vi "PWM Panel.vi"(8 "error in (no error)":errorcluster, 9 "PWM Configuration (\"\")":string, 10 "PWM Stimulus":T3={"Zero"=FALSE, "Blank Screen"=FALSE, "Offset"=FALSE, "Offset Value"=4.0, "Frequency (MHz)"=0.0}, 11 "PWM Command":T1=enum."MEASURE") -> (0 "error out":errorcluster, 1 "Variant Output":string, 2 "PWM Measurement":T2 caption="This reading is always in the base units\ni.e. V, A, Ohms, Hz, Sec, etc." format="%#_10f")   [LabVIEW 2011]
uses:
  PWM Measurement.ctl
  PWM Parameters.ctl
  PWM Command.ctl
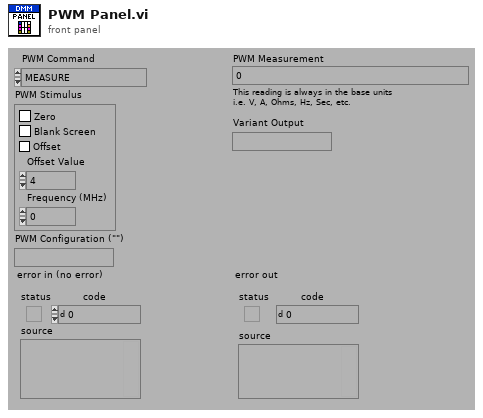
[diagram p1: front panel]
types:
  T1 = typedef "PWM Command.ctl" = enum16{"LOAD", "INITIALIZE", "PRESET", "GET STIMULUS", "SET STIMULUS", "MEASURE", "RELEASE", "UNLOAD", "GET CALIBRATION", "CALIBRATE"}
  T2 = typedef "PWM Measurement.ctl" = dbl
  T3 = typedef "PWM Parameters.ctl" = cluster{"Zero":bool, "Blank Screen":bool, "Offset":bool, "Offset Value":dbl, "Frequency (MHz)":dbl}
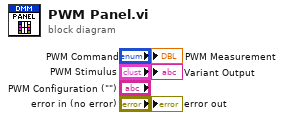
[diagram p0: block diagram]
diagram:
